vi "Documentation.vi"   [LabVIEW 2019, in "Inst.MOTOR.lvclass"]
uses:
  Inst.MOTOR.lvclass
  f6f46be3-8c07-4c28-bc0e-69594390ac78.vi
  9169cc93-ed84-4232-9f90-6ee16c7bb454.vi
  de41cf0e-ff2b-4a51-852c-55dbec0e345b.vi
  f6f46be3-8c07-4c28-bc0e-69594390ac78.vi/1d947704-3031-4246-b6a5-a3dbf98f6dfa.vi
  <userlib>/LevyLab/Instrument Framework/SMOs/Instrument/API/Send and Receive.vi
  f6f46be3-8c07-4c28-bc0e-69594390ac78.vi/e868c17e-0726-4176-ad7c-864f147f3c28.vi
  <userlib>/LevyLab/Instrument Framework/SMOs/Instrument/Private/Get Client Type.vi
  9169cc93-ed84-4232-9f90-6ee16c7bb454.vi/c2ec44ee-2e7a-4cb3-8659-4ccead6ee9ca.vi
  de41cf0e-ff2b-4a51-852c-55dbec0e345b.vi/482a3fd0-6f8c-4a9a-8993-9f11321ba70f.vi
  f6f46be3-8c07-4c28-bc0e-69594390ac78.vi/1d947704-3031-4246-b6a5-a3dbf98f6dfa.vi/a68c65c3-cc50-4065-8d6d-354ebbae477d.vi
  f6f46be3-8c07-4c28-bc0e-69594390ac78.vi/1d947704-3031-4246-b6a5-a3dbf98f6dfa.vi/4e227151-abc0-4d2a-aa4b-ce6c5f4112b0.vi
  f6f46be3-8c07-4c28-bc0e-69594390ac78.vi/e868c17e-0726-4176-ad7c-864f147f3c28.vi/54ef750c-c051-4a9e-95ed-99534d3d4017.vi
  f6f46be3-8c07-4c28-bc0e-69594390ac78.vi/e868c17e-0726-4176-ad7c-864f147f3c28.vi/e1955c45-aced-43f7-8a06-39fa822cb770.vi
  9169cc93-ed84-4232-9f90-6ee16c7bb454.vi/c2ec44ee-2e7a-4cb3-8659-4ccead6ee9ca.vi/b734b2bc-fc6e-447b-9123-2ba62aff1649.vi
  9169cc93-ed84-4232-9f90-6ee16c7bb454.vi/c2ec44ee-2e7a-4cb3-8659-4ccead6ee9ca.vi/51999fd1-8dee-42e4-abc3-5007bea80533.vi
  de41cf0e-ff2b-4a51-852c-55dbec0e345b.vi/482a3fd0-6f8c-4a9a-8993-9f11321ba70f.vi/8373d337-cfd8-4b11-b3e4-8c8651b39cee.vi
  de41cf0e-ff2b-4a51-852c-55dbec0e345b.vi/482a3fd0-6f8c-4a9a-8993-9f11321ba70f.vi/83ced2ad-04fd-4bef-a436-11c4aa46a55e.vi
  f6f46be3-8c07-4c28-bc0e-69594390ac78.vi/e868c17e-0726-4176-ad7c-864f147f3c28.vi/54ef750c-c051-4a9e-95ed-99534d3d4017.vi/e0fe7e29-4bd2-4ad2-a27b-9b2fd57412dc.vi
  f6f46be3-8c07-4c28-bc0e-69594390ac78.vi/e868c17e-0726-4176-ad7c-864f147f3c28.vi/54ef750c-c051-4a9e-95ed-99534d3d4017.vi/b2f436dc-64a0-41bb-9a2d-680b360754ee.vi
  9169cc93-ed84-4232-9f90-6ee16c7bb454.vi/c2ec44ee-2e7a-4cb3-8659-4ccead6ee9ca.vi/b734b2bc-fc6e-447b-9123-2ba62aff1649.vi/7d9fd4d2-9209-4cc8-ae8a-a6e5747f8095.vi
  9169cc93-ed84-4232-9f90-6ee16c7bb454.vi/c2ec44ee-2e7a-4cb3-8659-4ccead6ee9ca.vi/b734b2bc-fc6e-447b-9123-2ba62aff1649.vi/21f44e7a-1407-4f2f-b6bc-8a4269c4b59e.vi
  9169cc93-ed84-4232-9f90-6ee16c7bb454.vi/c2ec44ee-2e7a-4cb3-8659-4ccead6ee9ca.vi/51999fd1-8dee-42e4-abc3-5007bea80533.vi/9823380c-67ba-42a6-9007-75a1911aaea2.vi
  9169cc93-ed84-4232-9f90-6ee16c7bb454.vi/c2ec44ee-2e7a-4cb3-8659-4ccead6ee9ca.vi/51999fd1-8dee-42e4-abc3-5007bea80533.vi/6b1f7437-d69b-4163-8fbe-7b994795127e.vi
  de41cf0e-ff2b-4a51-852c-55dbec0e345b.vi/482a3fd0-6f8c-4a9a-8993-9f11321ba70f.vi/8373d337-cfd8-4b11-b3e4-8c8651b39cee.vi/217de07b-6c2e-4153-9c38-5f6facf85015.vi
  de41cf0e-ff2b-4a51-852c-55dbec0e345b.vi/482a3fd0-6f8c-4a9a-8993-9f11321ba70f.vi/8373d337-cfd8-4b11-b3e4-8c8651b39cee.vi/54b607cb-a4a3-4be3-aba5-75e0c970c1b7.vi
  de41cf0e-ff2b-4a51-852c-55dbec0e345b.vi/482a3fd0-6f8c-4a9a-8993-9f11321ba70f.vi/83ced2ad-04fd-4bef-a436-11c4aa46a55e.vi/d591628e-765d-47d5-9b6e-592bb07122c4.vi
  de41cf0e-ff2b-4a51-852c-55dbec0e345b.vi/482a3fd0-6f8c-4a9a-8993-9f11321ba70f.vi/83ced2ad-04fd-4bef-a436-11c4aa46a55e.vi/a50a5c75-8ad2-4065-a55b-fffdeda1dd49.vi
  9169cc93-ed84-4232-9f90-6ee16c7bb454.vi/c2ec44ee-2e7a-4cb3-8659-4ccead6ee9ca.vi/51999fd1-8dee-42e4-abc3-5007bea80533.vi/9823380c-67ba-42a6-9007-75a1911aaea2.vi/f6a6fdc4-833f-42ba-a963-d60e8082fc04.vi
  9169cc93-ed84-4232-9f90-6ee16c7bb454.vi/c2ec44ee-2e7a-4cb3-8659-4ccead6ee9ca.vi/51999fd1-8dee-42e4-abc3-5007bea80533.vi/9823380c-67ba-42a6-9007-75a1911aaea2.vi/d45465f2-7e5d-4c43-80cb-e663b9bd9eea.vi
  de41cf0e-ff2b-4a51-852c-55dbec0e345b.vi/482a3fd0-6f8c-4a9a-8993-9f11321ba70f.vi/83ced2ad-04fd-4bef-a436-11c4aa46a55e.vi/d591628e-765d-47d5-9b6e-592bb07122c4.vi/b0889090-0888-4513-91e6-1e5abe182f9c.vi
  de41cf0e-ff2b-4a51-852c-55dbec0e345b.vi/482a3fd0-6f8c-4a9a-8993-9f11321ba70f.vi/83ced2ad-04fd-4bef-a436-11c4aa46a55e.vi/d591628e-765d-47d5-9b6e-592bb07122c4.vi/51d16b6c-259f-4465-a302-1a6be0003813.vi
  <userlib>/LevyLab/Instrument Framework/SMOs/Instrument/Private/Get RC Connection Status.vi
  <userlib>/LevyLab/Instrument Framework/SMOs/Instrument/API/Enum to String.vi
  <userlib>/LevyLab/Instrument Framework/SMOs/RemoteControl/API/Send and Receive.vi
  <vilib>/Utility/Data Type/Get Type Information.vi
  <vilib>/JDP Science/JSONtext/JSON text to Variant.vi
  <vilib>/JDP Science/JSONtext/Variant to JSON Text.vi
  <vilib>/National Instruments/GUID Generator/Guid Generator.vi
  <userlib>/LevyLab/Instrument Framework/SMOs/Instrument/Private/Instrument.MessageFromProcess.EventStructure.vi
  <userlib>/LevyLab/Instrument Framework/SMOs/Instrument/Instrument.lvclass
  <vilib>/JKI/JKI SMO/SMO/SMO.lvclass
  Typedefs/Inst.MOTOR.getAll--Cluster.ctl
  Typedefs/Inst.MOTOR.Commands--Enum.ctl
  Inst UI.MOTOR/Inst UI.MOTOR.lvclass
  Inst UI.MOTOR/Inst UI.MOTOR.UI--Cluster.ctl
  <userlib>/LevyLab/Instrument Framework/SMOs/Instrument UI/Instrument UI.lvclass
  <vilib>/JKI/JKI SMO/SMO.UI/SMO.UI.lvclass
  Typedefs/Inst.MOTOR.Configuration--Cluster.ctl
  <vilib>/JDP Science/JSONtext/LVClass Serializer/JSONtext LVClass Serializer.lvclass
  <userlib>/LevyLab/Instrument Framework/SMOs/RemoteControl/RemoteControl.lvclass
  C:/Program Files (x86)/National Instruments/LabVIEW 2019/vi.lib/JKI/JKI SMO/SMO/SMO.lvclass
  C:/Program Files (x86)/National Instruments/LabVIEW 2019/user.lib/LevyLab/Instrument Framework/SMOs/Instrument/Instrument.lvclass
  C:/Program Files (x86)/National Instruments/LabVIEW 2019/user.lib/LevyLab/Instrument Framework/SMOs/Instrument UI/Instrument UI.lvclass
  C:/Program Files (x86)/National Instruments/LabVIEW 2019/vi.lib/JKI/JKI SMO/SMO.UI/SMO.UI.lvclass
types:
  T1 = typedef "Inst.MOTOR.lvclass/Inst.MOTOR.getAll--Cluster.ctl" = cluster{"Response":string, "Forward":bool, "Stop Motor":bool, "Encoder Position":string}
  T2 = typedef "Inst.MOTOR.lvclass/Inst.MOTOR.Commands--Enum.ctl" = enum16{"Encoder Position", "VISA Read", "VISA Write"}
  T3 = typedef "Inst.MOTOR.lvclass/Inst.MOTOR.Configuration--Cluster.ctl" = cluster{"baud rate":u32, "data bits":u16, "parity":enum16{"None", "Odd", "Even", "Mark", "Space"}, "stop bits":u16, "flow control":u16, "Read Count":u32, "Address":refnum<visa-resource-name>, "Termination Character":u8}
  T4 = typedef "Inst UI.MOTOR.lvclass/Inst UI.MOTOR.UI--Cluster.ctl" = cluster{" Read":string, "VISA resource name":refnum<visa-resource-name>}
  T5 = typedef "Instrument.lvclass/PublicEvents--Cluster.ctl" = cluster{"MessageFromProcess":refnum<user-event>}
  T6 = typedef "Instrument.lvclass/PrivateEvents--Cluster.ctl" = cluster{"MessageToProcess":refnum<user-event>, "Log PGSQL":refnum<user-event>}
  T7 = typedef "Inst.MOTOR.lvclass/PublicEvents--Cluster.ctl" = cluster{"MessageFromProcess":refnum<user-event>}
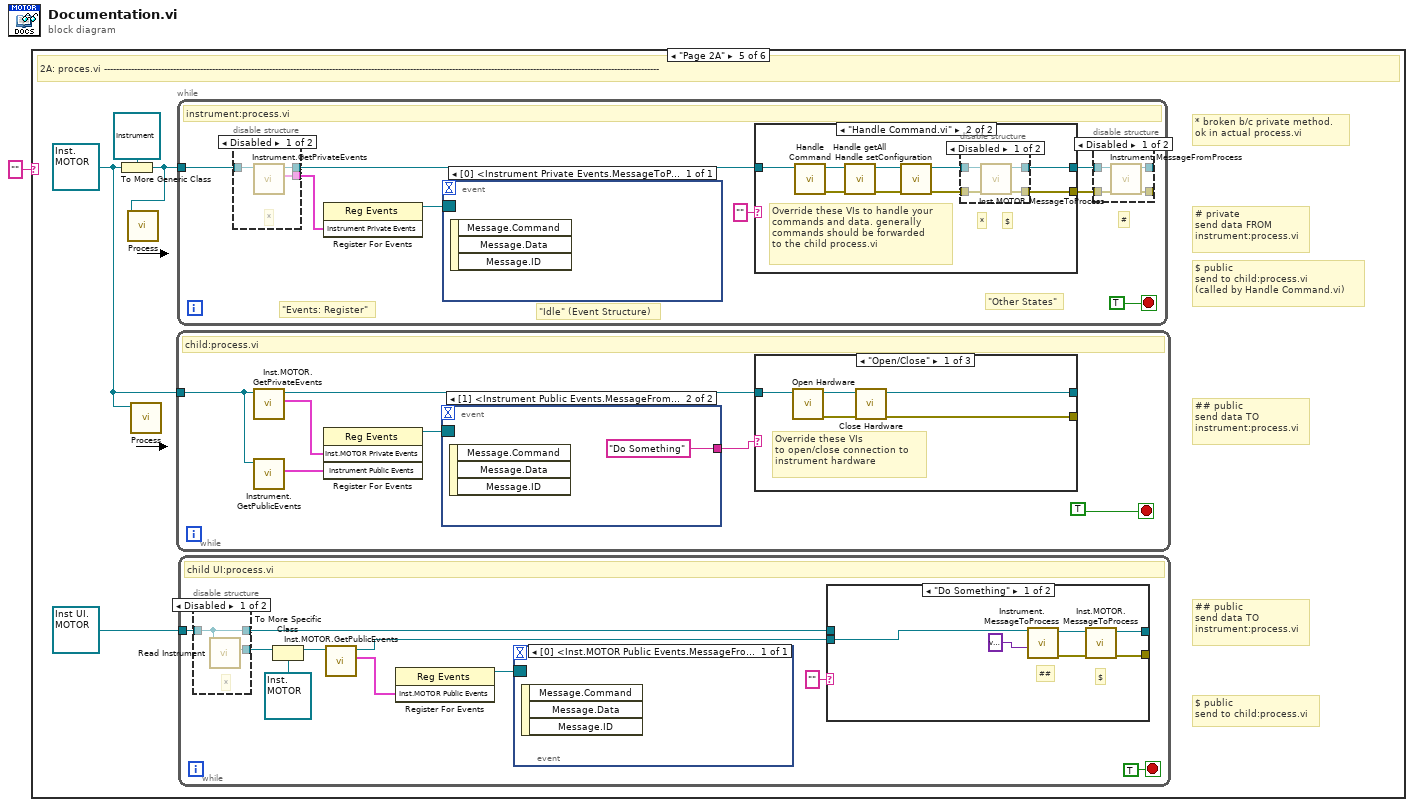
[diagram p0: block diagram]
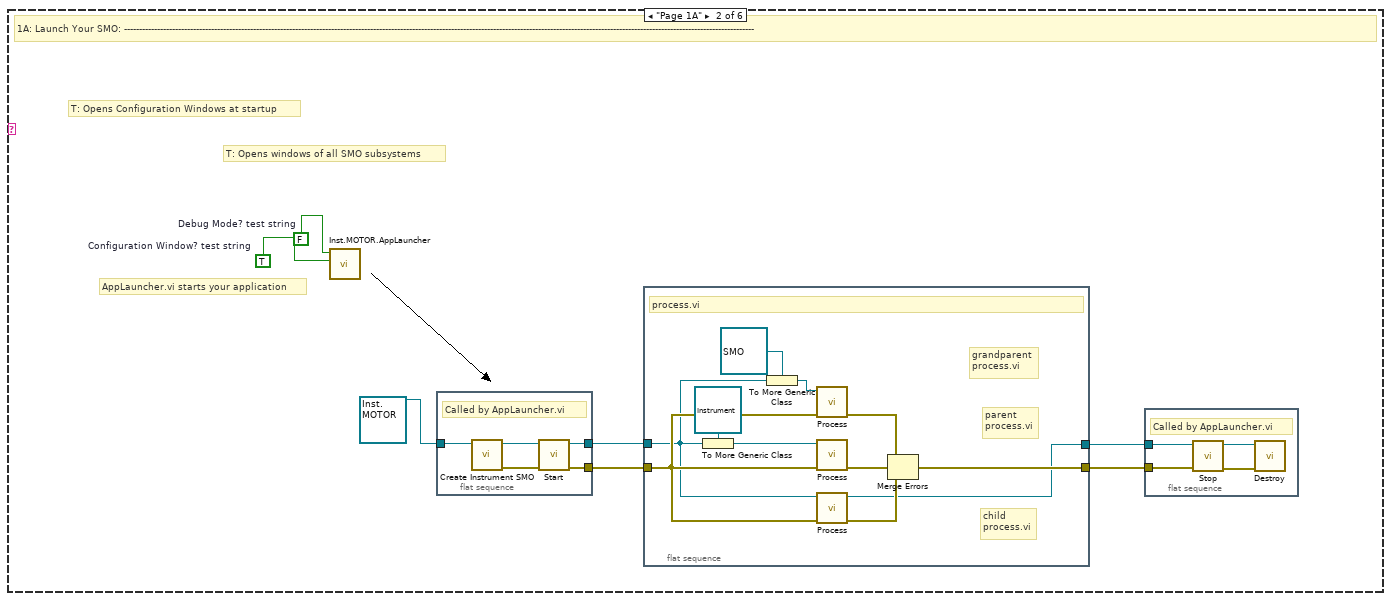
[diagram p3: hidden frame]
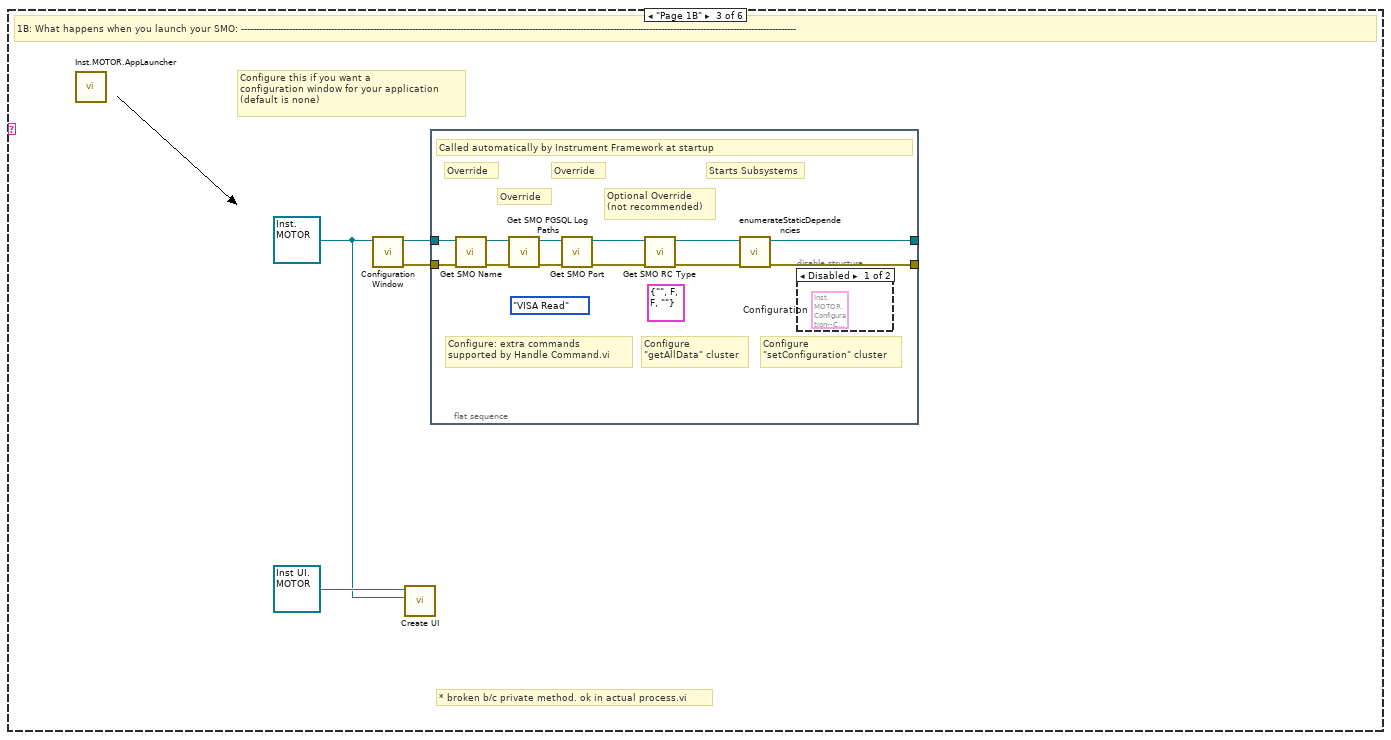
[diagram p4: hidden frame]
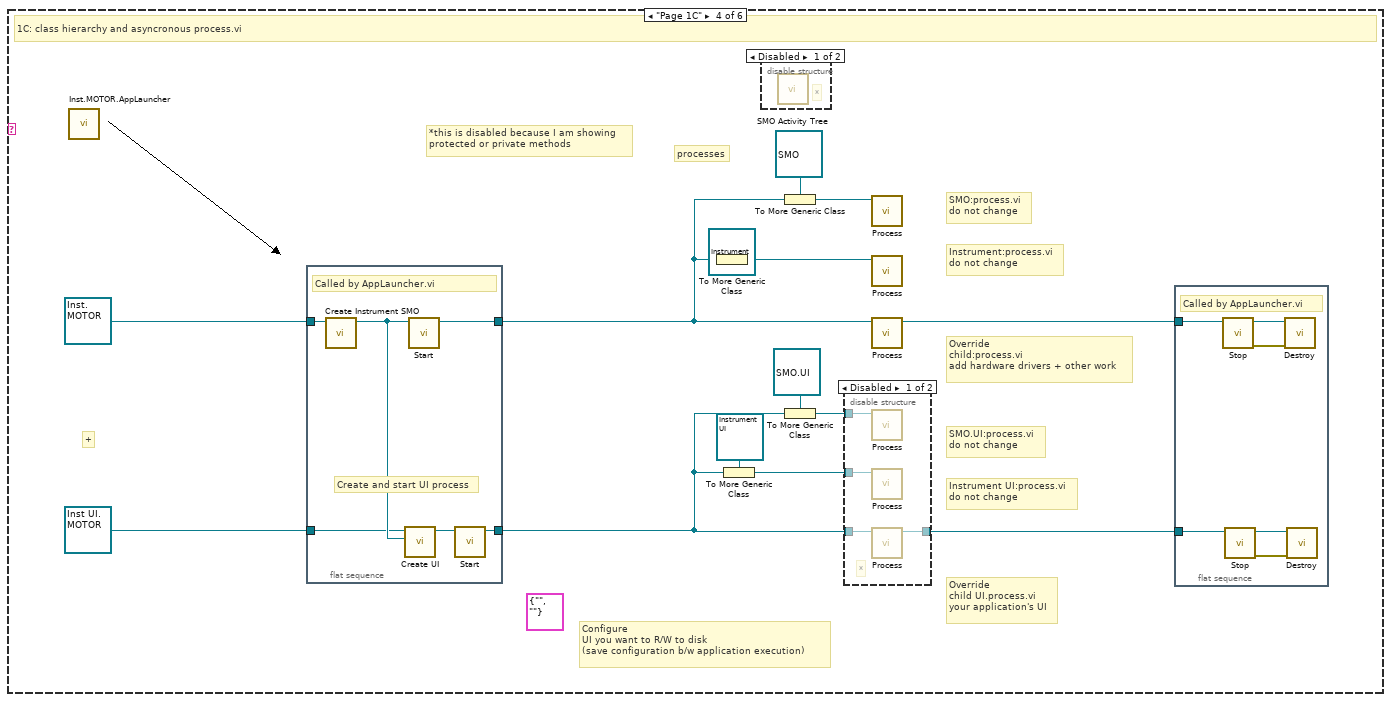
[diagram p6: hidden frame]
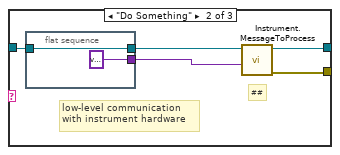
[diagram p11: hidden frame]
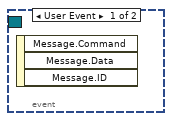
[diagram p13: hidden frame]
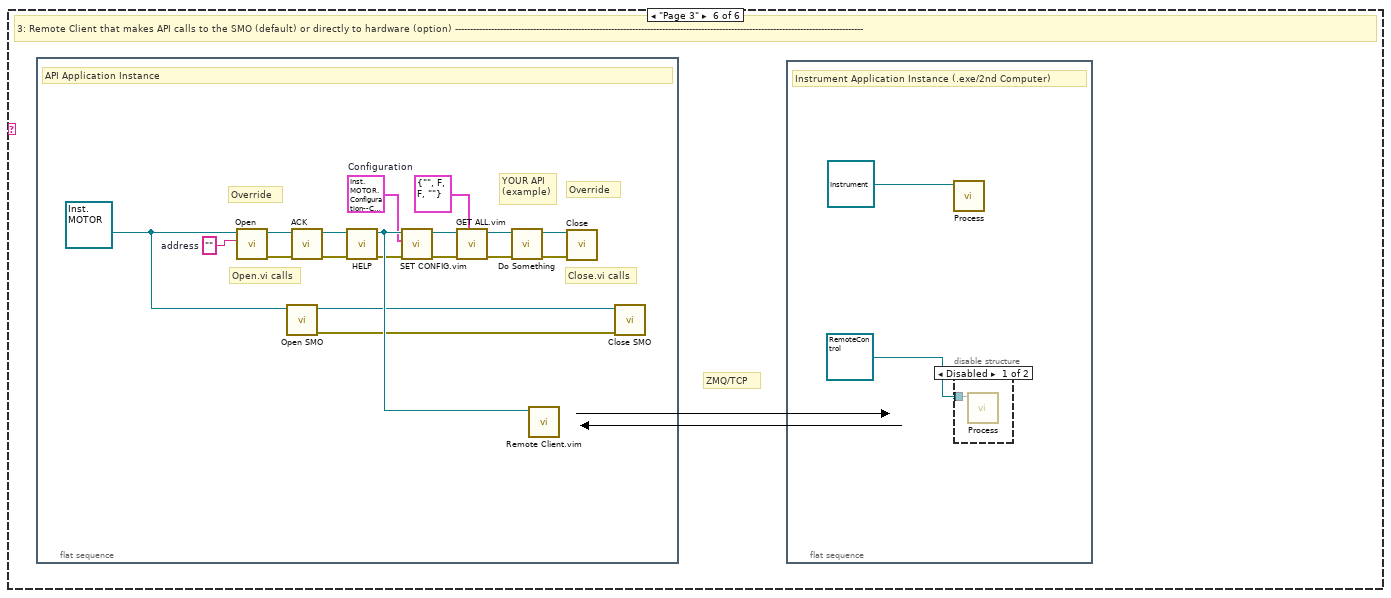
[diagram p18: hidden frame]
diagram:
  n1 = case shown="\"Page 2A\"" "" {
    frame Default {
    }
    frame "Page 1A" {
      w7 = TRUE  # Configuration Window? test string
      w8 = FALSE  # Debug Mode? test string
      # "AppLauncher.vi starts your application"
      # "T: Opens windows of all SMO subsystems"
      # "T: Opens Configuration Windows at startup"
      # "1A: Launch Your SMO: ------------------------------------------------------------------------------------------------------------------------------------------------------------------------------------------------------------------"
      n2 = call "Inst.MOTOR.AppLauncher.vi"("Config Window"=w7, "Debug Mode"=w8) -> ()  [unwired: 9 in, 1 out]
      n3 = flat-sequence {
        tunnel: [w26] -> w3
        tunnel: [w25] -> w5
        tunnel: refnum<class "Inst.MOTOR.lvclass"> refnum ("Instrument.Template.lvclass") -> [w24]
        frame #0 {
          # "Called by AppLauncher.vi"
          n4 = call-dynamic "Create Instrument SMO.vi"("Instrument in"=w24) -> ("error out"=w27:errorcluster, "Instrument out"=w28:refnum<class "Inst.MOTOR.lvclass">)  [unwired: 9 in]
          n5 = call <vilib>:"Start.vi"("error in (no error)"=w27, "SMO"=w28) -> ("error out"=w25:errorcluster, "SMO out"=w26:refnum<class "Inst.MOTOR.lvclass">)  [unwired: 8 in]
        }
      }
      n6 = flat-sequence {
        tunnel: [w19] -> w6
        tunnel: w5 -> [w17]
        tunnel: [w11] -> w4
        tunnel: w3 -> [w10]
        frame #0 {
          # "child\nprocess.vi"
          # "grandparent\nprocess.vi"
          # "parent\nprocess.vi"
          # "process.vi"
          n7 = To More Generic Class(target class=refnum<class "Instrument.lvclass"> refnum ("Instrument"), reference=w10) -> (generic class reference=w16:refnum<class "Instrument.lvclass">)
          n8 = To More Generic Class(target class=refnum<class "SMO.lvclass"> refnum ("SMO"), reference=w10) -> (generic class reference=w18:refnum<class "SMO.lvclass">)
          n9 = call-dynamic "Process.vi"("error in"=w17, "SMO"=w18) -> ("error out"=w12:errorcluster)  [unwired: 8 in, 1 out]
          n10 = call-dynamic "Process.vi"("error in"=w17, "Instrument"=w16) -> ("error out"=w14:errorcluster)  [unwired: 8 in, 1 out]
          n11 = call-dynamic "Process.vi"("error in"=w17, "Inst.MOTOR"=w10) -> ("error out"=w13:errorcluster, "Inst.MOTOR out"=w11:refnum<class "Inst.MOTOR.lvclass">)  [unwired: 8 in]
          n12 = Merge Errors(w12, w14, w13) -> (w19:errorcluster)
        }
      }
      n13 = flat-sequence {
        tunnel: w4 -> [w21]
        tunnel: w6 -> [w20]
        frame #0 {
          # "Called by AppLauncher.vi"
          n14 = call <vilib>:"Stop.vi"("error in (no error)"=w20, "SMO"=w21) -> ("error out"=w23:errorcluster, "SMO out"=w22:refnum<class "Inst.MOTOR.lvclass">)  [unwired: 8 in]
          n15 = call <vilib>:"Destroy.vi"("error in (no error)"=w23, "SMO"=w22) -> ()  [unwired: 9 in, 1 out]
        }
      }
    }
    frame "Page 1B" {
      w29 = refnum<class "Inst.MOTOR.lvclass"> refnum ("Instrument.Template.lvclass")
      # "* broken b/c private method. ok in actual process.vi"
      # "Configure this if you want a\nconfiguration window for your application\n(default is none)"
      # "1B: What happens when you launch your SMO: -----------------------------------------------------------------------------------------------------------------------------------------------------------------------------------------"
      n16 = call "Inst.MOTOR.AppLauncher.vi"() -> ()  [unwired: 11 in, 1 out]
      n17 = call-dynamic "Configuration Window.vi"("Inst.MOTOR in"=w29) -> ("error out"=w31:errorcluster, "Inst.MOTOR out"=w32:refnum<class "Inst.MOTOR.lvclass">)  [unwired: 9 in]
      n18 = call <userlib>:"Create UI.vi"("Instrument in"=w29, "Instrument UI"=refnum<class "Inst UI.MOTOR.lvclass"> refnum ("Instrument UI.Template.lvclass")) -> ()  [unwired: 8 in, 2 out]
      n19 = flat-sequence {
        tunnel: w32 -> [w40]
        tunnel: w31 -> [w35]
        tunnel: [w34] -> _
        tunnel: [w33] -> _
        frame #0 {
          (unwired) Inst.MOTOR.Commands--Enum."VISA Read" ("Commands")
          (unwired) T1 {"Response"="", "Forward"=FALSE, "Stop Motor"=FALSE, "Encoder Position"=""} ("getAll")
          # "Configure\n\"setConfiguration\" cluster"
          # "Configure\n\"getAllData\" cluster"
          # "Configure: extra commands\nsupported by Handle Command.vi"
          # "Starts Subsystems"
          # "Override"
          # "Override"
          # "Override"
          # "Optional Override\n(not recommended)"
          # "Called automatically by Instrument Framework at startup"
          n20 = call-dynamic "Get SMO Name.vi"("error in (no error)"=w35, "Inst.MOTOR in"=w40) -> ("error out"=w38:errorcluster, "Inst.MOTOR out"=w39:refnum<class "Inst.MOTOR.lvclass">)  [unwired: 7 in, 1 out]
          n21 = call-dynamic "Get SMO PGSQL Log Paths.vi"("error in (no error)"=w38, "Inst.MOTOR in"=w39) -> ("error out"=w36:errorcluster, "Inst.MOTOR out"=w37:refnum<class "Inst.MOTOR.lvclass">)  [unwired: 7 in, 1 out]
          n22 = call-dynamic "Get SMO Port.vi"("error in (no error)"=w36, "Inst.MOTORInstrument in"=w37) -> ("error out"=w41:errorcluster, "Inst.MOTORInstrument out"=w42:refnum<class "Inst.MOTOR.lvclass">)  [unwired: 7 in, 1 out]
          n23 = call-dynamic "Get SMO RC Type.vi"("error in (no error)"=w41, "Inst.MOTORInstrument in"=w42) -> ("error out"=w43:errorcluster, "Inst.MOTORInstrument out"=w44:refnum<class "Inst.MOTOR.lvclass">)  [unwired: 7 in, 1 out]
          n24 = call-dynamic "enumerateStaticDependencies.vi"("error in (no error)"=w43, "Instrument"=w44) -> ("error out"=w34:errorcluster, "Instrument out"=w33:refnum<class "Inst.MOTOR.lvclass">)  [unwired: 7 in, 1 out]
          n25 = disable-structure shown="Disabled" {
            frame Disabled {
              (unwired) T3 {"baud rate"=115200, "data bits"=8, "parity"=enum."None", "stop bits"=10, "flow control"=0, "Read Count"=1000, "Address"="COM3", "Termination Character"=10}  # Configuration
            }
            frame Enabled {
            }
          }
        }
      }
    }
    frame "Page 1C" {
      (unwired) T4 {" Read"="", "VISA resource name"=""} ("UI")
      # "processes"
      # "SMO.UI:process.vi\ndo not change"
      # "Instrument UI:process.vi\ndo not change"
      # "Override\nchild:process.vi\nadd hardware drivers + other work"
      # "SMO:process.vi\ndo not change"
      # "Instrument:process.vi\ndo not change"
      # "*this is disabled because I am showing\nprotected or private methods"
      # "Configure\nUI you want to R/W to disk\n(save configuration b/w application execution)"
      # "Override\nchild UI.process.vi\nyour application's UI"
      # "+"
      # "1C: class hierarchy and asyncronous process.vi"
      n26 = call "Inst.MOTOR.AppLauncher.vi"() -> ()  [unwired: 11 in, 1 out]
      n27 = flat-sequence {
        tunnel: [w74] -> w57
        tunnel: refnum<class "Inst.MOTOR.lvclass"> refnum ("Instrument.Template.lvclass") -> [w73]
        tunnel: refnum<class "Inst UI.MOTOR.lvclass"> refnum ("Instrument UI.Template.lvclass") -> [w71]
        tunnel: [w69] -> w55
        frame #0 {
          # "Create and start UI process"
          # "Called by AppLauncher.vi"
          n28 = call-dynamic "Create Instrument SMO.vi"("Instrument in"=w73) -> ("Instrument out"=w72:refnum<class "Inst.MOTOR.lvclass">)  [unwired: 9 in, 1 out]
          n29 = call <userlib>:"Create UI.vi"("Instrument in"=w72, "Instrument UI"=w71) -> ("Instrument UI out"=w70:refnum<class "Inst UI.MOTOR.lvclass">)  [unwired: 8 in, 1 out]
          n30 = call <vilib>:"Start.vi"("SMO"=w72) -> ("SMO out"=w74:refnum<class "Inst.MOTOR.lvclass">)  [unwired: 9 in, 1 out]
          n31 = call <vilib>:"Start.vi"("SMO"=w70) -> ("SMO out"=w69:refnum<class "Inst UI.MOTOR.lvclass">)  [unwired: 9 in, 1 out]
        }
      }
      n32 = To More Generic Class(target class=refnum<class "Instrument.lvclass"> refnum ("Instrument"), reference=w57) -> (generic class reference=w52:refnum<class "Instrument.lvclass">)
      n33 = To More Generic Class(target class=refnum<class "Instrument UI.lvclass"> refnum ("Instrument UI"), reference=w55) -> (generic class reference=w48:refnum<class "Instrument UI.lvclass">)
      n34 = disable-structure shown="Disabled" {
        frame Disabled {
          # "*"
          n35 = call <vilib>:"SMO Activity Tree.vi"() -> ()  [unwired: 12 in]
        }
        frame Enabled {
        }
      }
      n36 = To More Generic Class(target class=refnum<class "SMO.lvclass"> refnum ("SMO"), reference=w57) -> (generic class reference=w53:refnum<class "SMO.lvclass">)
      n37 = To More Generic Class(target class=refnum<class "SMO.UI.lvclass"> refnum ("SMO.UI"), reference=w55) -> (generic class reference=w46:refnum<class "SMO.UI.lvclass">)
      n38 = disable-structure shown="Disabled" {
        disable-tunnel: w55 -> [w62 _]
        disable-tunnel: [w61 _] -> w54
        disable-tunnel: w48 -> [w60 _]
        disable-tunnel: w46 -> [w59 _]
        frame Disabled {
          # "*"
          n39 = call-dynamic "Process.vi"("SMO.UI"=w59) -> ()  [unwired: 9 in, 2 out]
          n40 = call-dynamic "Process.vi"("Instrument UI in"=w60) -> ()  [unwired: 9 in, 2 out]
          n41 = call-dynamic "Process.vi"("Inst UI.MOTOR"=w62) -> ("Inst UI.MOTOR out"=w61:refnum<class "Inst UI.MOTOR.lvclass">)  [unwired: 9 in, 1 out]
        }
        frame Enabled {
        }
      }
      n42 = call-dynamic "Process.vi"("SMO"=w53) -> ()  [unwired: 9 in, 2 out]
      n43 = call-dynamic "Process.vi"("Instrument"=w52) -> ()  [unwired: 9 in, 2 out]
      n44 = call-dynamic "Process.vi"("Inst.MOTOR"=w57) -> ("Inst.MOTOR out"=w58:refnum<class "Inst.MOTOR.lvclass">)  [unwired: 9 in, 1 out]
      n45 = flat-sequence {
        tunnel: w58 -> [w66]
        tunnel: w54 -> [w64]
        frame #0 {
          # "Called by AppLauncher.vi"
          n46 = call <vilib>:"Stop.vi"("SMO"=w66) -> ("error out"=w68:errorcluster, "SMO out"=w67:refnum<class "Inst.MOTOR.lvclass">)  [unwired: 9 in]
          n47 = call <vilib>:"Stop.vi"("SMO"=w64) -> ("error out"=w65:errorcluster, "SMO out"=w63:refnum<class "Inst UI.MOTOR.lvclass">)  [unwired: 9 in]
          n48 = call <vilib>:"Destroy.vi"("error in (no error)"=w68, "SMO"=w67) -> ()  [unwired: 9 in, 1 out]
          n49 = call <vilib>:"Destroy.vi"("error in (no error)"=w65, "SMO"=w63) -> ()  [unwired: 9 in, 1 out]
        }
      }
    }
    frame "Page 2A" {
      w75 = refnum<class "Inst.MOTOR.lvclass"> refnum ("Instrument.Template.lvclass")
      # "## public\nsend data TO\ninstrument:process.vi"
      # "$ public\nsend to child:process.vi"
      # "## public\nsend data TO\ninstrument:process.vi"
      # "$ public\nsend to child:process.vi\n(called by Handle Command.vi)"
      # "# private\nsend data FROM\ninstrument:process.vi"
      # "* broken b/c private method.\nok in actual process.vi"
      # "2A: proces.vi -----------------------------------------------------------------------------------------------------------------------------------------------------------------------------------------"
      n50 = To More Generic Class(target class=refnum<class "Instrument.lvclass"> refnum ("Instrument"), reference=w75) -> (generic class reference=w76:refnum<class "Instrument.lvclass">)
      n51 = call-dynamic "Process.vi"("Instrument"=w76) -> ()  [unwired: 9 in, 2 out]
      n52 = call-dynamic "Process.vi"("Inst.MOTOR"=w75) -> ()  [unwired: 9 in, 2 out]
      n53 = while {
        tunnel: w75 -> [w101]
        stop <- TRUE stop-if-true
        # "child:process.vi"
        n54 = call "Inst.MOTOR.GetPrivateEvents.vi"("Inst.MOTOR in"=w101) -> ("Inst.MOTOR Private Events"=w105:cluster{"MessageToProcess":refnum<user-event>}, "Inst.MOTOR out"=w103:refnum<class "Inst.MOTOR.lvclass">)  [unwired: 8 in, 1 out]
        n55 = call <userlib>:"Instrument.GetPublicEvents.vi"("Instrument"=w101) -> ("Instrument Public Events"=w102:T5)  [unwired: 8 in, 2 out]
        n56 = register-events(w105, w102) -> (reference out=w104:refnum<event-registration>)  [unwired: 2 in, 1 out]
        n57 = event shown="[1] <Instrument Public Events.MessageFromProcess>: User Event" {
          selector: w104 -> [_ _]
          dyn-events: _ -> [_ _]
          timeout: _ -> [_ _]
          tunnel: [_ "Do Something"] -> w99
          event User Event {
            n58 = event-data() -> ()  [unwired: 1 in, 3 out]
          }
          event User Event {
            n59 = event-data() -> ()  [unwired: 1 in, 3 out]
          }
        }
        n60 = case shown="\"Open/Close\"" w99 {
          tunnel: w103 -> [w108 w113 w118]
          tunnel: [w107 w115 w118] -> _
          tunnel: [w106 w114 _] -> _
          frame "Open/Close" {
            # "Override these VIs\nto open/close connection to\ninstrument hardware"
            n61 = call-dynamic "Open Hardware.vi"("Inst.MOTOR in"=w108) -> ("error out"=w110:errorcluster, "Inst.MOTOR out"=w109:refnum<class "Inst.MOTOR.lvclass">)  [unwired: 9 in]
            n62 = call-dynamic "Close Hardware.vi"("error in (no error)"=w110, "Inst.MOTOR in"=w109) -> ("error out"=w106:errorcluster, "Inst.MOTOR out"=w107:refnum<class "Inst.MOTOR.lvclass">)  [unwired: 8 in]
          }
          frame "Do Something" {
            # "##"
            # "low-level communication\nwith instrument hardware"
            n63 = flat-sequence {
              tunnel: w113 -> [w117]
              tunnel: [w117] -> w112
              tunnel: [variant ("Data")] -> w111
              frame #0 {
              }
            }
            n64 = call <userlib>:"Instrument.MessageToProcess.vi"("Data"=w111, "Instrument"=w112) -> ("error out"=w114:errorcluster, "Instrument out"=w115:refnum<class "Inst.MOTOR.lvclass">)  [unwired: 8 in]
          }
          frame Default {
          }
        }
      }
      n65 = while {
        tunnel: w76 -> [w126]
        stop <- TRUE stop-if-true
        # "#"
        # "\"Other States\""
        # "\"Idle\" (Event Structure)"
        # "\"Events: Register\""
        # "instrument:process.vi"
        n66 = disable-structure shown="Disabled" {
          disable-tunnel: w126 -> [w150 w151]
          disable-tunnel: [w149 w151] -> w125
          disable-tunnel: [w148 _] -> w124
          frame Disabled {
            # "*"
            n67 = call <userlib>:"Instrument.GetPrivateEvents.vi"("Instrument"=w150) -> ("Instrument Private Events"=w148:T6, "Instrument out"=w149:refnum<class "Instrument.lvclass">)  [unwired: 8 in, 1 out]
          }
          frame Enabled {
          }
        }
        n68 = register-events(w124) -> (reference out=w123:refnum<event-registration>)  [unwired: 2 in, 1 out]
        n69 = event shown="[0] <Instrument Private Events.MessageToProcess>: User Event" {
          selector: w123 -> [_]
          dyn-events: _ -> [_]
          timeout: _ -> [_]
          event User Event {
            n70 = event-data() -> ()  [unwired: 1 in, 3 out]
          }
        }
        n71 = case shown="\"Handle Command.vi\"" "" {
          tunnel: w125 -> [w132 w141]
          tunnel: [w132 w135] -> w122
          tunnel: [_ w134] -> w121
          frame Default {
          }
          frame "Handle Command.vi" {
            # "*"
            # "$"
            # "Override these VIs to handle your\ncommands and data. generally \ncommands should be forwarded\nto the child process.vi"
            n72 = call-dynamic "Handle Command.vi"("Instrument in"=w141) -> ("error out"=w137:errorcluster, "Instrument out"=w140:refnum<class "Instrument.lvclass">)  [unwired: 7 in, 2 out]
            n73 = call-dynamic "Handle getAll.vi"("error in (no error)"=w137, "Instrument in"=w140) -> ("error out"=w138:errorcluster, "Instrument out"=w139:refnum<class "Instrument.lvclass">)  [unwired: 7 in, 1 out]
            n74 = call-dynamic "Handle setConfiguration.vi"("error in (no error)"=w138, "Instrument in"=w139) -> ("error out"=w133:errorcluster, "Instrument out"=w136:refnum<class "Instrument.lvclass">)  [unwired: 8 in]
            n75 = disable-structure shown="Disabled" {
              disable-tunnel: w136 -> [w145 w147]
              disable-tunnel: [w144 w147] -> w135
              disable-tunnel: [w143 w146] -> w134
              disable-tunnel: w133 -> [w142 w146]
              frame Disabled {
                n76 = call "Inst.MOTOR.MessageToProcess.vi"("error in (no error)"=w142, "Inst.MOTOR in"=w145) -> ("error out"=w143:errorcluster, "Inst.MOTOR out"=w144:refnum<class "Inst.MOTOR.lvclass">)  [unwired: 8 in]
              }
              frame Enabled {
              }
            }
          }
        }
        n77 = disable-structure shown="Disabled" {
          disable-tunnel: w122 -> [w131 _]
          disable-tunnel: w121 -> [w130 _]
          disable-tunnel: [w129 _] -> _
          disable-tunnel: [w128 _] -> _
          frame Disabled {
            n78 = call <userlib>:"Instrument.MessageFromProcess.vi"("error in (no error)"=w130, "Instrument"=w131) -> ("error out"=w129:errorcluster, "Instrument out"=w128:refnum<class "Instrument.lvclass">)  [unwired: 8 in]
          }
          frame Enabled {
          }
        }
      }
      n79 = while {
        tunnel: refnum<class "Inst UI.MOTOR.lvclass"> refnum ("Instrument UI.Template.lvclass") -> [w87]
        stop <- TRUE stop-if-true
        # "child UI:process.vi"
        n80 = disable-structure shown="Disabled" {
          disable-tunnel: w87 -> [w96 w98]
          disable-tunnel: [w97 _] -> w85
          disable-tunnel: [w96 w98] -> w81
          frame Disabled {
            # "*"
            n81 = call <userlib>:"Read Instrument.vi"("Instrument UI in"=w96) -> ("Instrument"=w97:refnum<class "Instrument.lvclass">)  [unwired: 8 in, 2 out]
          }
          frame Enabled {
          }
        }
        n82 = To More Specific Class(target class=refnum<class "Inst.MOTOR.lvclass"> refnum ("Instrument.Template.lvclass"), reference=w85) -> (specific class reference=w84:refnum<class "Inst.MOTOR.lvclass">)  [unwired: 1 in, 1 out]
        n83 = call "Inst.MOTOR.GetPublicEvents.vi"("Inst.MOTOR in"=w84) -> ("Inst.MOTOR Public Events"=w82:T7, "Inst.MOTOR out"=w80:refnum<class "Inst.MOTOR.lvclass">)  [unwired: 8 in, 1 out]
        n84 = register-events(w82) -> (reference out=w83:refnum<event-registration>)  [unwired: 2 in, 1 out]
        n85 = event shown="[0] <Inst.MOTOR Public Events.MessageFromProcess>: User Event" {
          selector: w83 -> [_]
          dyn-events: _ -> [_]
          timeout: _ -> [_]
          event User Event {
            n86 = event-data() -> ()  [unwired: 1 in, 3 out]
          }
        }
        n87 = case shown="\"Do Something\"" "" {
          tunnel: w81 -> [_ _]
          tunnel: [w91 w95] -> _
          tunnel: [w90 _] -> _
          tunnel: w80 -> [w92 w95]
          frame "Do Something" {
            # "##"
            # "$"
            n88 = call <userlib>:"Instrument.MessageToProcess.vi"("Data"=variant, "Instrument"=w92) -> ("error out"=w89:errorcluster, "Instrument out"=w93:refnum<class "Inst.MOTOR.lvclass">)  [unwired: 8 in]
            n89 = call "Inst.MOTOR.MessageToProcess.vi"("error in (no error)"=w89, "Inst.MOTOR in"=w93) -> ("error out"=w90:errorcluster, "Inst.MOTOR out"=w91:refnum<class "Inst.MOTOR.lvclass">)  [unwired: 8 in]
          }
          frame Default {
          }
        }
      }
    }
    frame "Page 3" {
      # "ZMQ/TCP"
      # "3: Remote Client that makes API calls to the SMO (default) or directly to hardware (option) ----------------------------------------------------------------------------------------------------------------------------------------"
      n90 = flat-sequence {
        frame #0 {
          w157 = ""  # address
          w162 = T3 {"baud rate"=0, "data bits"=0, "parity"=enum."None", "stop bits"=10, "flow control"=0, "Read Count"=1000, "Address"="", "Termination Character"=10}  # Configuration
          w172 = refnum<class "Inst.MOTOR.lvclass"> refnum ("Instrument.Template.lvclass")
          # "Close.vi calls"
          # "Open.vi calls"
          # "YOUR API\n(example)"
          # "Override"
          # "Override"
          # "API Application Instance"
          n91 = call-dynamic "Open.vi"("address"=w157, "Inst.MOTOR in"=w172) -> ("error out"=w170:errorcluster, "Inst.MOTOR out"=w169:refnum<class "Inst.MOTOR.lvclass">)  [unwired: 8 in]
          n92 = call <userlib>:"Open SMO.vi"("Instrument in"=w172) -> ("error out"=w155:errorcluster, "Instrument out"=w156:refnum<class "Inst.MOTOR.lvclass">)  [unwired: 9 in]
          n93 = call <userlib>:"ACK.vi"("error in (no error)"=w170, "Instrument in"=w169) -> ("error out"=w168:errorcluster, "Instrument out"=w167:refnum<class "Inst.MOTOR.lvclass">)  [unwired: 7 in, 1 out]
          n94 = call <userlib>:"HELP.vi"("error in (no error)"=w168, "Instrument in"=w167) -> ("error out"=w163:errorcluster, "Instrument in"=w171:refnum<class "Inst.MOTOR.lvclass">)  [unwired: 7 in, 1 out]
          n95 = call "SET CONFIG.vim"("error in (no error)"=w163, "Configuration"=w162, "Instrument in"=w171) -> ("error out"=w158:errorcluster, "Instrument out"=w161:refnum<class "Inst.MOTOR.lvclass">)  [unwired: 7 in]
          n96 = call "GET ALL.vim"("type"=T1 {"Response"="", "Forward"=FALSE, "Stop Motor"=FALSE, "Encoder Position"=""} ("getAll"), "error in (no error)"=w158, "Instrument in"=w161) -> ("error out"=w159:errorcluster, "Instrument out"=w160:refnum<class "Inst.MOTOR.lvclass">)  [unwired: 6 in, 1 out]
          n97 = call-dynamic "Do Something.vi"("error in (no error)"=w159, "Inst.MOTOR in"=w160) -> ("error out"=w165:errorcluster, "Inst.MOTOR out"=w166:refnum<class "Inst.MOTOR.lvclass">)  [unwired: 8 in]
          n98 = call "Remote Client.vim"("Instrument in"=w171) -> ()  [unwired: 7 in, 4 out]
          n99 = call-dynamic "Close.vi"("error in (no error)"=w165, "Inst.MOTOR in"=w166) -> ()  [unwired: 8 in, 2 out]
          n100 = call <userlib>:"Close SMO.vi"("error in (no error)"=w155, "Instrument in"=w156) -> ()  [unwired: 8 in, 2 out]
        }
      }
      n101 = flat-sequence {
        frame #0 {
          # "Instrument Application Instance (.exe/2nd Computer)"
          n102 = call-dynamic "Process.vi"("Instrument"=refnum<class "Instrument.lvclass"> refnum) -> ()  [unwired: 9 in, 2 out]
          n103 = disable-structure shown="Disabled" {
            disable-tunnel: refnum<class "RemoteControl.lvclass"> refnum ("RemoteControl out") -> [w154 _]
            frame Disabled {
              n104 = call-dynamic "Process.vi"("RemoteControl"=w154) -> ()  [unwired: 9 in, 2 out]
            }
            frame Enabled {
            }
          }
        }
      }
    }
  }
